vi "MathCad_Matrix_Insert_to_Wrksht.vi"(3 "error out 2":errorcluster, 4 "New Variable Name":string, 5 "Mathcad.IMatrixValue Reference In":refnum<k7>, 6 "Worksheet Reference In":refnum<k7>) -> (0 "error out":errorcluster, 1 "Mathcad.IMatrixValue Reference Out":refnum<k7>, 2 "Worksheet Reference Out":refnum<k7>)   [LabVIEW 2015]
doc: "Inserts value into the worksheet. This has to be done after the value has been set for the worksheet to recieve the new value."
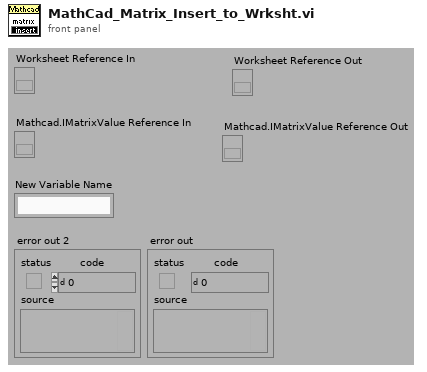
[diagram p1: front panel]
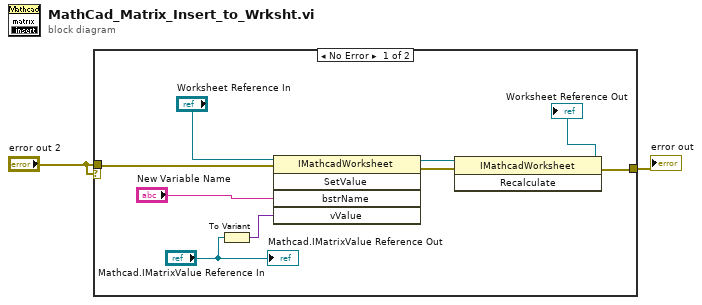
[diagram p0: block diagram]
diagram:
  n1 = case shown="No Error" "error out 2" {
    tunnel: [w3 w12] -> w2
    tunnel: "error out 2" -> [w10 w12]
    frame No Error {
      n2 = To Variant(anything="Mathcad.IMatrixValue Reference In") -> (Variant=w8:variant)
      n3 = invoke class="IMathcadWorksheet" method="SetValue"(reference="Worksheet Reference In", error in=w10, "bstrName"="New Variable Name", "vValue"=w8) -> (reference out=w6:refnum<k7>, error out=w5:errorcluster)  [unwired: 1 in, 3 out]
      n4 = invoke class="IMathcadWorksheet" method="Recalculate"(reference=w6, error in=w5) -> (reference out=→"Worksheet Reference Out":refnum<k7>, error out=w3:errorcluster)  [unwired: 1 in, 1 out]
      "Mathcad.IMatrixValue Reference Out" <- "Mathcad.IMatrixValue Reference In"
    }
    frame Error {
    }
  }
  "error out" <- w2
